vi "Add.vi"(2 "AngleAdd":refnum<class "Angle.lvclass">, 3 "Angle in":refnum<class "Angle.lvclass">) -> (0 "Output":dbl, 1 "?":refnum<class "Angle.lvclass">)   [LabVIEW 2013, in "Angle.lvclass"]
doc: "Bonnie Ishiguro, Fall 2013\n\nTakes two angles as inputs and returns their sum."
uses:
  Angle.lvclass
  Angle.lvclass/Angle.ctl
panel:
  in  "Angle out":refnum<class "Angle.lvclass">
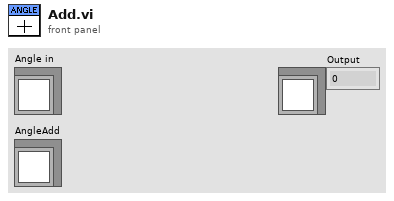
[diagram p1: front panel]
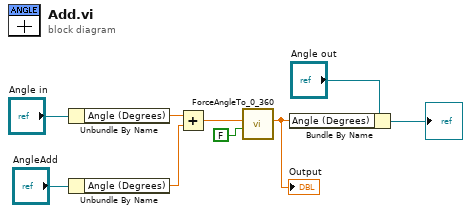
[diagram p0: block diagram]
diagram:
  n1 = Unbundle By Name("Angle in") -> ("Angle (Degrees)"=w8:dbl)
  n2 = Unbundle By Name("AngleAdd") -> ("Angle (Degrees)"=w6:dbl)
  n3 = Add(x=w8, y=w6) -> (x+y=w3:dbl)
  n4 = call "ForceAngleTo_0_360.vi"("Use angle class? (T)"=FALSE, "Angle in"=w3) -> ("Forced Angle"=w2:dbl)  [unwired: 7 in, 2 out]
  "Output" <- w2
  n5 = Bundle By Name(cluster="Angle out", "Angle (Degrees)"=w2) -> (→"?":refnum<class "Angle.lvclass">)
